vi "_MDPtr Validate DataFrame Type.vi"(7 "error in (no error)":errorcluster, 9 "Data Type":T1, 10 "data":T2) -> (0 "error out":errorcluster, 3 "data (dup)":T2)   [LabVIEW 2014]
uses:
  MDPtr TypeDef/MDPtr.ctl
  MDPtr TypeDef/MDPtr SupportedDataTypeDef.ctl
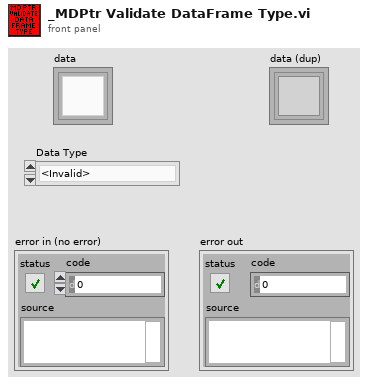
[diagram p1: front panel]
types:
  T1 = typedef "MDPtr SupportedDataTypeDef.ctl" = enum16{"<Invalid>", "Waveform", "Waveform Arr", "Double Arr"}
  T2 = typedef "MDPtr.ctl" = refnum<k1>
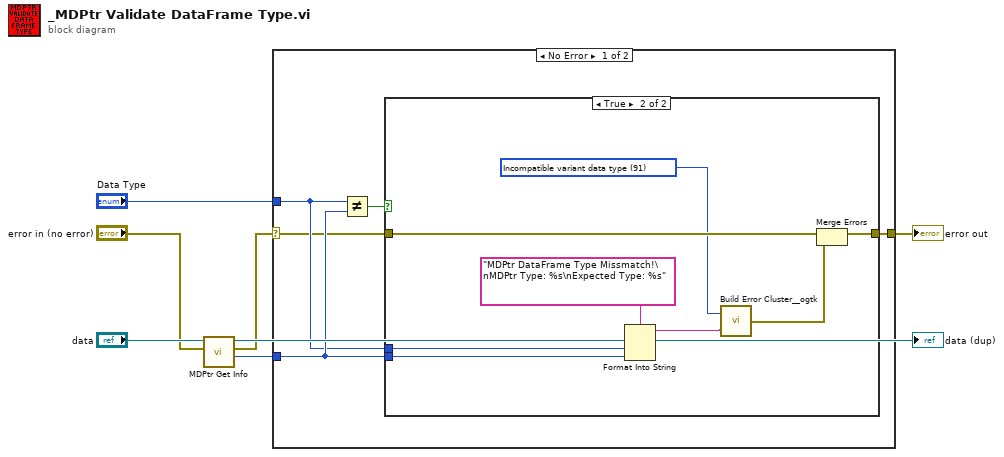
[diagram p0: block diagram]
diagram:
  n1 = call "MDPtr Get Info.vi"("error in (no error)"="error in (no error)", "HexStrPtr"="data") -> ("Data Type"=w4:T1, "error out"=w1:errorcluster, "HexStrPtr (dup)"=→"data (dup)":T2)  [unwired: 5 in, 1 out]
  n2 = case shown="No Error" w1 {
    selector: w1 -> [w8 w22]
    tunnel: [w12 w22] -> w7
    tunnel: w4 -> [w10 _]
    tunnel: "Data Type" -> [w9 _]
    frame No Error {
      n3 = Not Equal?(x=w9, y=w10) -> (x != y?=w11:bool)
      n4 = case shown="True" w11 {
        tunnel: [w13 w21] -> w12
        tunnel: w8 -> [w13 w20]
        tunnel: w10 -> [_ w18]
        tunnel: w9 -> [_ w19]
        frame False {
        }
        frame True {
          w14 = 91 items=["No error", "Argument error", "Memory is full", "Out of zone", "End of file", "File already open", "Generic file I/O error", "File not found", "File permission error", "Disk is full", "Duplicate path", "Too many files open", "System feature not enabled", "Resource file not found", "Cannot add resource", "Resource not found", "Image not found", "Image memory error", "Pen does not exist", "Config type invalid", "Config token not found", "Config parse error", "Config memory error", "Bad external code format", "Bad external code offset", "External code not present", "Null window", "Destroy window error", "Null menu", "Print aborted", "Bad print record", "Print driver error", "Windows error during printing", "Memory error during printing", "Print dialog error", "Generic print error", "Invalid device refnum", "Device not found", "Device parameter error", "Device unit error", "Cannot open device", "Device call aborted", "Generic error", "Cancelled by user", "Object ID too low", "Object ID too high", "Object not in heap", "Unknown heap", "Unknown object (invalid DefProc)", "Unknown object (DefProc not in table)", "Message out of range", "Invalid (null) method", "Unknown message", "Manager call not supported", "Bad address", "Network operation in progress", "Network operation timed out", "Connection is busy", "Network attribute not supported", "Network error", "Address in use", "System out of memory", "Connection aborted", "Connection refused", "Not connected", "Already connected", "Connection closed", "Initialization error (interapplication manager)", "Bad occurrence", "Wait on unbound occurrence handler", "Occurrence queue overflow", "Datalog type conflict", "Unused", "Unrecognized type (interapplication manager)", "Memory corrupt", "Failed to make temporary DLL", "Old CIN version", "Drag socket not found", "Failed to load drop-object", "Failed to register OLE object", "Failed to release OLE object", "Format specifier type mismatch", "Unknown format specifier", "Too few format specifiers", "Too many format specifiers", "Scan failed", "Newer CIN version", "Error converting to variant", "Runtime menu error", "Password tampered", "Variant attribute not found", "Incompatible variant data type", "Event data is not available", "Event Store is not present", "Occurrence is not found", "Event Queue is not created", "Event info is not available", "Refnum passed is NULL", "Error retrieving Class GUID", "Error retrieving CoClass GUID", "Error retrieving TypeLib GUID.", "Bad built application magic bytes.", "Specific driver is different from the specific driver associated with the Logical Name.", "There is no session opened to the class driver.", "Max Error", "MAX - Error with config objects", "MAX - Error loading configuration", "MAX - Group not supported"]
          n5 = Format Into String(format string="MDPtr DataFrame Type Missmatch!\nMDPtr Type: %s\nExpected Type: %s", w19, w18) -> (resulting string=w16:string)  [unwired: 2 in, 1 out]
          n6 = call <userlib>:"Build Error Cluster__ogtk.vi"("String to Prepend to source (\"\")"=w16, "code"=w14) -> ("error out"=w15:errorcluster)
          n7 = Merge Errors(w20, w15) -> (w21:errorcluster)
        }
      }
    }
    frame Error {
    }
  }
  "error out" <- w7
